vi "AES Decrypt.vi"   [LabVIEW 2021, in "dotNET Crypto Symmetric Encryption.lvlib"]
doc: "Decrypt data using AES encryption. ECB and CBC block cipher modes are supported. ECB is considered cryptographically insecure and should not be used."
uses:
  dotNET Crypto Symmetric Encryption.lvlib
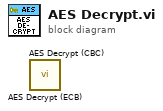
[diagram p0: block diagram]
diagram:
  n1 = call "AES Decrypt (ECB).vi"() -> ()  [unwired: 10 in, 2 out]
  n2 = call "AES Decrypt (CBC).vi"() -> ()  [unwired: 10 in, 2 out]
